vi "Intake Controller.vi"(8 "error in":errorcluster) -> ()   [LabVIEW 2019]
doc: "This VI executes continuously carrying out the current operation and responding to updates or new operations. It will often contain the timing or control code that is difficult to place directly in TeleOp. This VI generally opens all sensors and motors and isolates the rest of the robot code from knowing how the operations are carried out."
uses:
  <vilib>/Rock Robotics/WPI/Framework/Completion Status.ctl
  Intake Setpoints.ctl
  Intake Operations.ctl
  <vilib>/Rock Robotics/WPI/SafetyOutput/WPI_SafetyOutputConfigMenu.ctl
  <vilib>/Rock Robotics/WPI/Solenoid/WPI_SolenoidChannel.ctl
  <vilib>/Rock Robotics/WPI/Solenoid/WPI_SolenoidValue.ctl
  <vilib>/Rock Robotics/WPI/Solenoid/WPI_SolenoidOpenDouble.vi
  <vilib>/Rock Robotics/WPI/Solenoid/WPI_SolenoidSetEnum.vi
  <vilib>/Rock Robotics/WPI/Solenoid/WPI_SolenoidGetEnum.vi
  <vilib>/Rock Robotics/Network Tables/NT Write Boolean.vi
panel:
  in  "Interactive Values":T1
  out "Current\nCmd":string
  in  "Buttons":cluster{"Execute Cmd":bool, "Abort Cmd":bool}
  out "Command Timing":cluster{"Start Time (ms)":u32, "Iterations":i32}
  out "Status":T3
  # "Tip: It may be helpful to observe inputs and sensor values.\nYou may also want to display tuning or debugging controls."
  # "Interactive Command: You may fill in the settings for a command\nand schedule it with the Execute button. You can observe and abort\nany command while fine tuning the code for the controller."
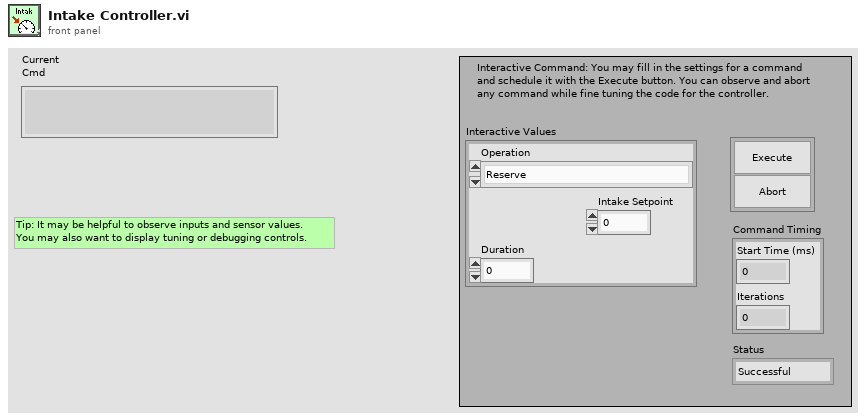
[diagram p1: front panel]
types:
  T1 = typedef "Intake Setpoints.ctl" = cluster{"Operation":T2, "Duration":dbl, "Intake Setpoint":dbl}
  T2 = typedef "Intake Operations.ctl" = enum16{"Reserve", "Read Current", "Immediate", "Change Intake State"}
  T3 = typedef "Completion Status.ctl" = enum16{"Successful", "Aborted", "Incomplete"}
  T4 = typedef "WPI_SolenoidValue.ctl" = enum16{"Off", "On", "Forward", "Reverse"}
  T5 = typedef "WPI_SolenoidChannel.ctl" = enum8{"Solenoid 0", "Solenoid 1", "Solenoid 2", "Solenoid 3", "Solenoid 4", "Solenoid 5", "Solenoid 6", "Solenoid 7", "Invalid"}
  T6 = typedef "WPI_SafetyOutputConfigMenu.ctl" = enum16{"Enable", "Disable"}
  T7 = typedef "WPI_MotorControlDeviceRef.ctl" = cluster{"DeviceStatus":errorcluster, "Type":T8, "PWM":cluster{"PWM Channel":T9, "DeadBand":T10}, "CAN":cluster{"Device Number":u8, "SetOutput VI Ref":variant, "GetOutput VI Ref":variant, "Enable VI Ref":variant, "Disable VI Ref":variant, "Data":variant}, "Invert":bool, "DIO PWM":cluster{"PWM \"Enable\" Channel":T9, "DIOChannel":T11, "PWM Rate":dbl}}
  T8 = typedef "WPI_MotorControlType.ctl" = enum16{"PWM", "CAN", "DIO PWM"}
  T9 = typedef "FPGA_DIOPWMChannel.ctl" = enum8{"PWM 0", "PWM 1", "PWM 2", "PWM 3", "PWM 4", "PWM 5", "PWM 6", "PWM 7", "PWM 8", "PWM 9", "PWM MXP 0", "PWM MXP 1", "PWM MXP 2", "PWM MXP 3", "PWM MXP 4", "PWM MXP 5", "PWM MXP 6", "PWM MXP 7", "PWM MXP 8", "PWM MXP 9", "Invalid"}
  T10 = typedef "WPI_PWMDeadband.ctl" = cluster{"Name":string, "maxPositivePwm":i32, "minPositivePwm":i32, "centerPwm":i32, "maxNegativePwm":i32, "minNegativePwm":i32, "angularRange":u16}
  T11 = typedef "FPGA_DIOChannel.ctl" = enum8{"DIO 0", "DIO 1", "DIO 2", "DIO 3", "DIO 4", "DIO 5", "DIO 6", "DIO 7", "DIO 8", "DIO 9", "DIO MXP 0", "DIO MXP 1", "DIO MXP 2", "DIO MXP 3", "DIO MXP 4", "DIO MXP 5", "DIO MXP 6", "DIO MXP 7", "DIO MXP 8", "DIO MXP 9", "DIO MXP 10", "DIO MXP 11", "DIO MXP 12", "DIO MXP 13", "DIO MXP 14", "DIO MXP 15", "SPI Port CS1", "SPI Port CS2", "SPI Port CS3", "SPI Port MISO", "SPI Port MOSI", "Invalid"}
  T12 = typedef "WPI_SolenoidDevRef.ctl" = cluster{"DevStatus":errorcluster, "Pneumatics Control Module":u8, "Forward Solenoid Channel":T5, "Reverse Solenoid Channel":T5}
  T13 = typedef "Command Status Info.ctl" = cluster{"Name":string, "Status":T3, "notifier out":T14}
  T14 = typedef "Completion Notifier.ctl" = refnum<notifier>
  T15 = cluster{"Current Command":T1, "Command Timing":cluster{"Start Time (ms)":u32, "Iterations":i32}, "Command Arguments":cluster{"Command Info":T13, "Description":string, "Default Command":T1, "queue out":refnum<queue>, "Subsystem Name":string}}
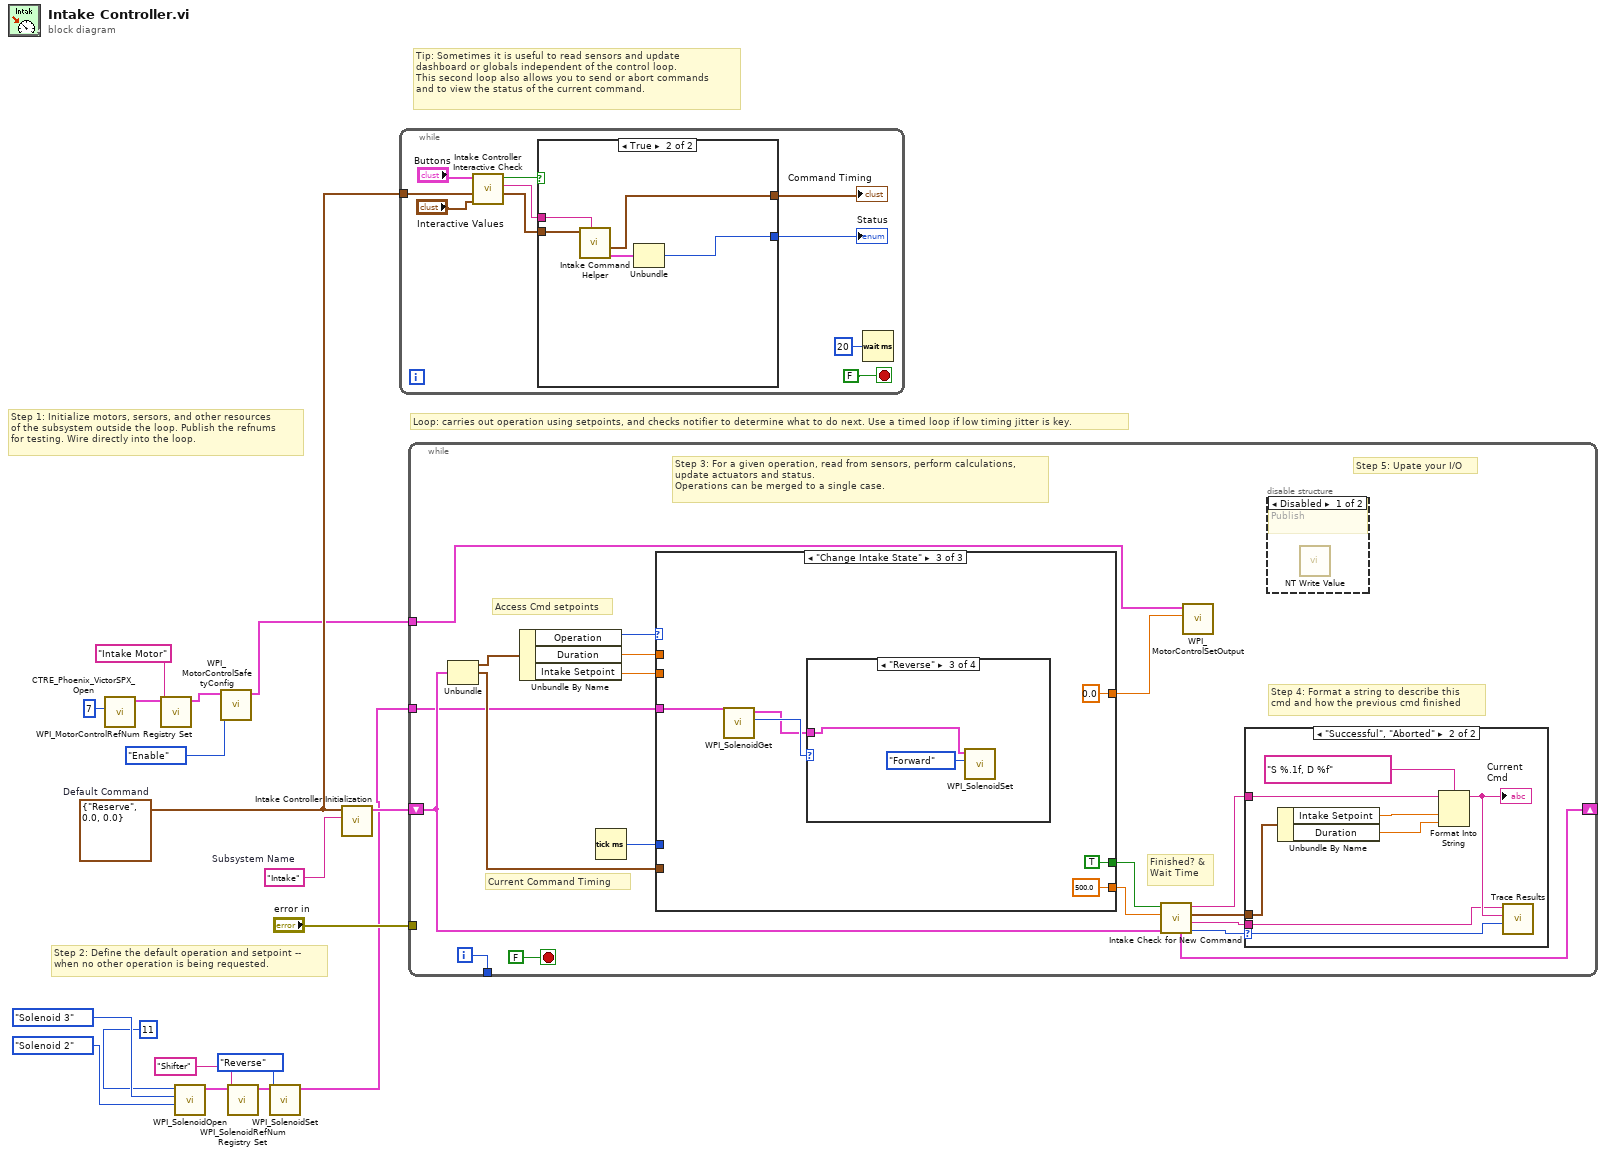
[diagram p0: block diagram]
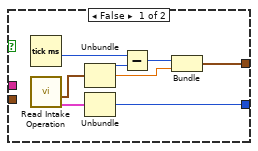
[diagram p2: hidden frame]
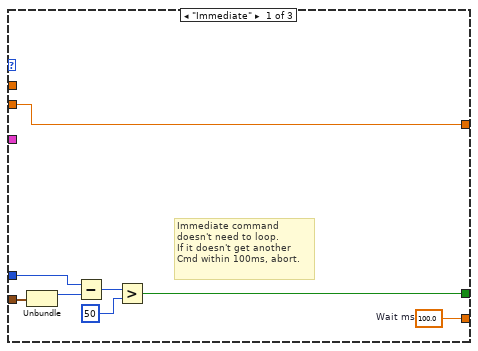
[diagram p5: hidden frame]
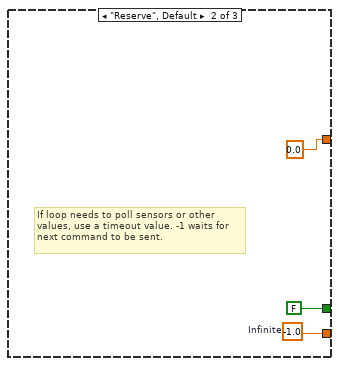
[diagram p6: hidden frame]
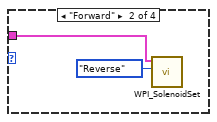
[diagram p8: hidden frame]
diagram:
  w15 = T1 {"Operation"=enum."Reserve", "Duration"=0.0, "Intake Setpoint"=0.0}  # Default Command
  w16 = "Intake"  # Subsystem Name
  # "Tip: Sometimes it is useful to read sensors and update\ndashboard or globals independent of the control loop.\nThis second loop also allows you to send or abort commands\nand to view the status of the current command."
  # "Step 2: Define the default operation and setpoint --\nwhen no other operation is being requested."
  # "Step 1: Initialize motors, sersors, and other resources\nof the subsystem outside the loop. Publish the refnums\nfor testing. Wire directly into the loop."
  # "Loop: carries out operation using setpoints, and checks notifier to determine what to do next. Use a timed loop if low timing jitter is key."
  n1 = call <vilib>:"CTRE_Phoenix_VictorSPX_Open.vi"("Device Number"=u8 7) -> ("CAN Talon SRX Ref"=w13:T7)  [unwired: 9 in, 1 out]
  n2 = call <vilib>:"WPI_MotorControlRefNum Registry Set.vi"("refnum name"="Intake Motor", "MotorControlDevRef"=w13) -> ("MotorControlDevRef"=w11:T7)  [unwired: 8 in, 1 out]
  n3 = call-poly <vilib>:"WPI_SolenoidOpen.vi"("Reverse Solenoid Channel"=WPI_SolenoidChannel."Solenoid 2", "Forward Solenoid Channel"=WPI_SolenoidChannel."Solenoid 3", "Pneumatics Control Module (0)"=11) -> ("SolenoidDevRef"=w5:T12)  [unwired: 7 in, 1 out]
  n4 = call <vilib>:"WPI_MotorControlSafetyConfig.vi"("mode"=WPI_SafetyOutputConfigMenu."Enable", "MotorControlDevRef"=w11) -> ("MotorControlDevRef"=w9:T7)  [unwired: 8 in, 1 out]
  n5 = call <vilib>:"WPI_SolenoidRefNum Registry Set.vi"("refnum name"="Shifter", "SolenoidDevRef"=w5) -> ("SolenoidDevRef"=w4:T12)  [unwired: 8 in, 1 out]
  n6 = call-poly <vilib>:"WPI_SolenoidSet.vi"("Value"=WPI_SolenoidValue."Reverse", "SolenoidDevRef"=w4) -> ("SolenoidDevRef"=w1:T12)  [unwired: 8 in, 1 out]
  n7 = call "Intake Controller Initialization.vi"("Subsystem Name"=w16, "Default Command"=w15) -> ("Current Command"=w17:T15)  [unwired: 9 in]
  n8 = while {
    tunnel: w15 -> [w25]
    stop <- FALSE stop-if-true
    n9 = call "Intake Controller Interactive Check.vi"("Interactive Command in"="Interactive Values", "Default Command"=w25, "Buttons"="Buttons") -> ("Interactive Command out"=w22:T1, "Trace String"=w23:string, "Schedule"=w24:bool)  [unwired: 6 in]
    n10 = case shown="True" w24 {
      tunnel: [w36 w41] -> w21
      tunnel: w22 -> [_ w39]
      tunnel: [w32 w37] -> w20
      tunnel: w23 -> [_ w40]
      frame False {
        n11 = Tick Count (ms)() -> (millisecond timer value=w31:u32)
        n12 = call "Read Intake Operation.vi"() -> ("Command Info"=w29:T13, "SubSystem Data"=w30:T1)  [unwired: 9 in, 1 out]
        n13 = Unbundle(w30) -> ("Operation"=w35:T2, "Duration"=w33:dbl)  [unwired: 1 out]
        n14 = Unbundle(w29) -> ("Status"=w36:T3)  [unwired: 2 out]
        n15 = Subtract(x=w31, y=w35) -> (x-y=w34:u32)
        n16 = Bundle(w34, "Duration"=w33) -> (w32:cluster{u32, "Duration":dbl})  [unwired: 1 in]
      }
      frame True {
        n17 = call "Intake Command Helper.vi"("Description"=w40, "SubSystem Data"=w39) -> ("Command Info Out"=w38:T13, "Command Timing"=w37:cluster{"Start Time (ms)":u32, "Iterations":i32})  [unwired: 7 in, 1 out]
        n18 = Unbundle(w38) -> ("Status"=w41:T3)  [unwired: 2 out]
      }
    }
    "Status" <- w21
    "Command Timing" <- w20
    n19 = Wait (ms)(milliseconds to wait=u32 20) -> ()  [unwired: 1 out]
  }
  n20 = while {
    shift-right: [w52] -> _
    shift-left: w17 -> [w45]
    tunnel: [w59] -> _
    tunnel: "error in" -> [_]
    tunnel: w9 -> [w43]
    tunnel: w1 -> [w42]
    i -> [w59]
    stop <- FALSE stop-if-true
    # "Step 5: Upate your I/O"
    # "Step 4: Format a string to describe this\ncmd and how the previous cmd finished"
    # "Current Command Timing"
    # "Access Cmd setpoints"
    # "Finished? &\nWait Time"
    # "Step 3: For a given operation, read from sensors, perform calculations,\nupdate actuators and status.\nOperations can be merged to a single case."
    n21 = Unbundle(w45) -> ("Current Command"=w58:T1, "Command Timing"=w54:cluster{"Start Time (ms)":u32, "Iterations":i32})  [unwired: 1 out]
    n22 = Unbundle By Name(w58) -> ("Operation"=w57:T2, "Duration"=w56:dbl, "Intake Setpoint"=w53:dbl)
    n23 = Tick Count (ms)() -> (millisecond timer value=w55:u32)
    n24 = case shown="\"Change Intake State\"" w57 {
      tunnel: [w76 w79 500.0 ("Infinite")] -> w50
      tunnel: [w70 FALSE ("ignore previous (F)") TRUE ("ignore previous (F)")] -> w51
      tunnel: w54 -> [w72 _ _]
      tunnel: w56 -> [_ _ _]
      tunnel: w55 -> [w71 _ _]
      tunnel: w53 -> [w69 _ _]
      tunnel: [w69 0.0 ("Setpoint") 0.0 ("Setpoint")] -> w44
      tunnel: w42 -> [_ _ w85]
      frame "Immediate" {
        w76 = 100.0  # Wait ms
        # "Immediate command\ndoesn't need to loop.\nIf it doesn't get another\nCmd within 100ms, abort."
        n25 = Unbundle(w72) -> ("Start Time (ms)"=w75:u32)  [unwired: 1 out]
        n26 = Subtract(x=w71, y=w75) -> (x-y=w74:u32)
        n27 = Greater?(x=w74, y=u8 50 ("Left Motor")) -> (0:w70:bool)
      }
      frame "Reserve", Default {
        w79 = -1.0  # Infinite
        # "If loop needs to poll sensors or other\nvalues, use a timeout value. -1 waits for\nnext command to be sent."
      }
      frame "Change Intake State" {
        n28 = call-poly <vilib>:"WPI_SolenoidGet.vi"("SolenoidDevRef"=w85) -> ("Value"=w84:T4, "SolenoidDevRef"=w83:T12)  [unwired: 8 in, 1 out]
        n29 = case shown="\"Reverse\"" w84 {
          tunnel: w83 -> [_ w87 w88 _]
          frame "Off", Default {
          }
          frame "Forward" {
            n30 = call-poly <vilib>:"WPI_SolenoidSet.vi"("Value"=WPI_SolenoidValue."Reverse", "SolenoidDevRef"=w87) -> ()  [unwired: 8 in, 2 out]
          }
          frame "Reverse" {
            n31 = call-poly <vilib>:"WPI_SolenoidSet.vi"("Value"=WPI_SolenoidValue."Forward", "SolenoidDevRef"=w88) -> ()  [unwired: 8 in, 2 out]
          }
          frame "On" {
          }
        }
      }
    }
    n32 = call "Intake Check for New Command.vi"("Current Command"=w45, "Wait time (ms)"=w50, "Finished?"=w51) -> ("Completion"=w46:T3, "Subsystem Name"=w47:string, "Current Command"=w48:T1, "Initial Trace String"=w49:string, "NextCommand"=w52:T15)  [unwired: 4 in]
    n33 = call <vilib>:"WPI_MotorControlSetOutput.vi"("Output"=w44, "MotorControlDevRef"=w43) -> ()  [unwired: 7 in, 3 out]
    n34 = case shown="\"Successful\", \"Aborted\"" w46 {
      selector: w46 -> [_ w68]
      tunnel: w49 -> [_ w64]
      tunnel: w48 -> [_ w65]
      tunnel: w47 -> [_ w61]
      frame "Incomplete", Default {
        # "Continuing current command"
      }
      frame "Successful", "Aborted" {
        # "Report and setup for next command"
        n35 = Unbundle By Name(w65) -> ("Intake Setpoint"=w67:dbl, "Duration"=w62:dbl)
        n36 = Format Into String(format string="S %.1f, D %f", initial string=w64, w67, w62) -> (resulting string=w63:string)  [unwired: 1 in, 1 out]
        "Current\nCmd" <- w63
        n37 = call <vilib>:"Trace Results.vi"("Status of previous command"=w68, "Description"=w63, "Subsystem"=w61) -> ()  [unwired: 9 in]
      }
    }
    n38 = disable-structure shown="Disabled" {
      frame Disabled {
        # "Publish"
        n39 = call-poly <vilib>:"NT Write Value.vi"() -> ()  [unwired: 11 in, 1 out]
      }
      frame Enabled {
      }
    }
  }
